vi "Mux I18xN to IQ.vi"(0 "i16xn in":fxp<+/-,18,1>[](array[numeric]), 5 "index":i32, 9 "input valid":bool[](array[boolean])) -> (4 "output":T1, 10 "output valid":bool)   [LabVIEW 2018, in "Lock-In Amplifier Example FPGA.lvlib"]
uses:
  Lock-In Amplifier Example FPGA.lvlib
  <instrlib>/_niInstr/DSP/v1/Shared/Public/IQ Data.ctl
  <instrlib>/_niInstr/DSP/v1/Shared/niInstr DSP v1 Shared.lvlib
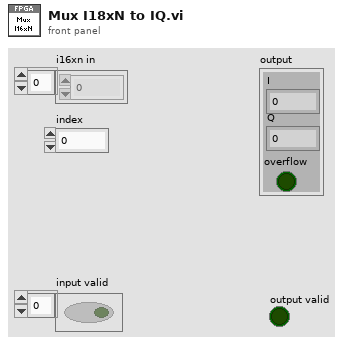
[diagram p1: front panel]
types:
  T1 = typedef "niInstr DSP v1 Shared.lvlib/IQ Data.ctl" = cluster{"I":fxp<+/-,18,1>, "Q":fxp<+/-,18,1>, "overflow":bool}
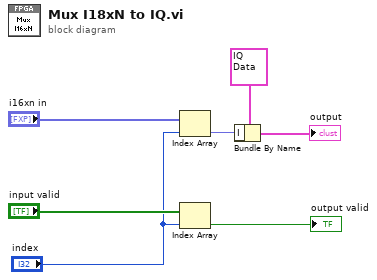
[diagram p0: block diagram]
diagram:
  n1 = Index Array(array="i16xn in", index="index") -> (element=w5:fxp<+/-,18,1>)
  n2 = Index Array(array="input valid", index="index") -> (element=→"output valid":bool)
  n3 = Bundle By Name(cluster=T1 {"I"=0.0, "Q"=0.0, "overflow"=FALSE} ("data"), "I"=w5) -> (→"output":T1)
